vi "Example2.2-FeedbackNode.vi"() -> ()   [LabVIEW 2019]
panel:
  out "Time Between Loop Iterations":dbl
  in  "ms to Wait":dbl=50.0
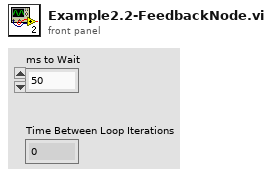
[diagram p1: front panel]
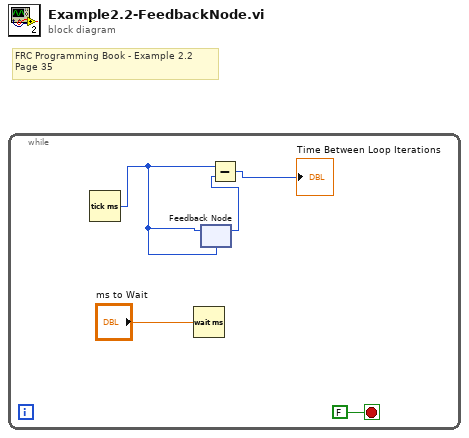
[diagram p0: block diagram]
diagram:
  # "FRC Programming Book - Example 2.2\nPage 35"
  n1 = while {
    stop <- FALSE stop-if-true
    n2 = Tick Count (ms)() -> (millisecond timer value=w2:u32)
    n3 = Wait (ms)(milliseconds to wait="ms to Wait") -> ()  [unwired: 1 out]
    n4 = feedback-in #1(w2) -> ()
    n5 = feedback #1(w2) -> (w1:u32)
    n6 = Subtract(x=w2, y=w1) -> (x-y=→"Time Between Loop Iterations":u32)
  }
